vi "TurnApprox.vi"(10 "Angle":dbl, 11 "RobotDriveDevRef":T1={"DevStatus"={"status"=FALSE, "code"=0, "source"=""}, "Motors[]"=[], "Square Inputs"=FALSE, "Max Output"=1.0}) -> (3 "RobotDriveDevRef":T1={"DevStatus"={"status"=FALSE, "code"=0, "source"=""}, "Motors[]"=[], "Square Inputs"=FALSE, "Max Output"=1.0})   [LabVIEW 2016]
uses:
  <vilib>/Rock Robotics/WPI/RobotDrive/WPI_RobotDriveDevRef.ctl
  <vilib>/Rock Robotics/WPI/MotorControl/WPI_MotorControlDeviceRef.ctl
  <vilib>/Rock Robotics/WPI/MotorControl/WPI_MotorControlType.ctl
  <vilib>/Rock Robotics/SystemInterfaces/DIO/FPGA_DIOPWMChannel.ctl
  <vilib>/Rock Robotics/WPI/PWM/WPI_PWMDeadband.ctl
  Robot Global Data.vi
  <vilib>/Rock Robotics/WPI/RobotDrive/WPI_RobotDriveArcadeDrive_Standard(NoSaturation).vi
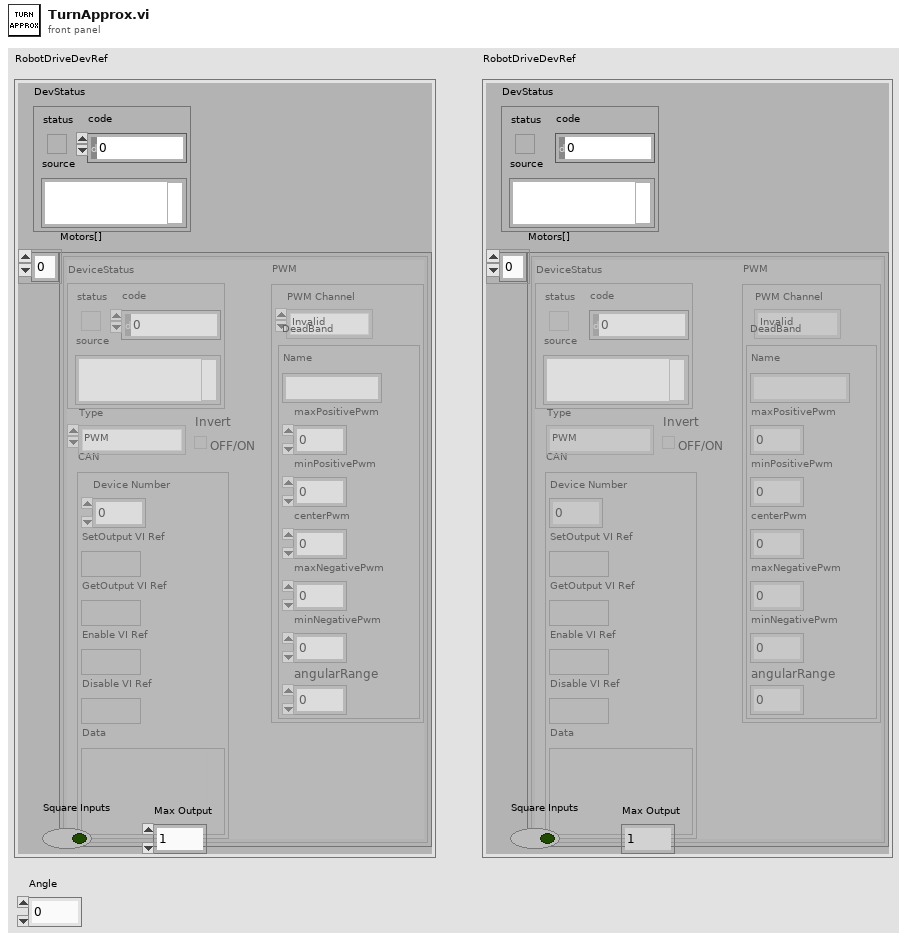
[diagram p1: front panel]
types:
  T1 = typedef "WPI_RobotDriveDevRef.ctl" = cluster{"DevStatus":errorcluster, "Motors[]":T2[], "Square Inputs":bool, "Max Output":dbl}
  T2 = typedef "WPI_MotorControlDeviceRef.ctl" = cluster{"DeviceStatus":errorcluster, "Type":T3, "PWM":cluster{"PWM Channel":T4, "DeadBand":T5}, "CAN":cluster{"Device Number":u8, "SetOutput VI Ref":variant, "GetOutput VI Ref":variant, "Enable VI Ref":variant, "Disable VI Ref":variant, "Data":variant}, "Invert":bool}
  T3 = typedef "WPI_MotorControlType.ctl" = enum16{"PWM", "CAN"}
  T4 = typedef "FPGA_DIOPWMChannel.ctl" = enum8{"PWM 0", "PWM 1", "PWM 2", "PWM 3", "PWM 4", "PWM 5", "PWM 6", "PWM 7", "PWM 8", "PWM 9", "PWM MXP 0", "PWM MXP 1", "PWM MXP 2", "PWM MXP 3", "PWM MXP 4", "PWM MXP 5", "PWM MXP 6", "PWM MXP 7", "PWM MXP 8", "PWM MXP 9", "Invalid"}
  T5 = typedef "WPI_PWMDeadband.ctl" = cluster{"Name":string, "maxPositivePwm":i32, "minPositivePwm":i32, "centerPwm":i32, "maxNegativePwm":i32, "minNegativePwm":i32, "angularRange":u16}
  T6 = cluster{"Lower X":dbl, "Lower Y":dbl, "Upper X":dbl, "Upper Y":dbl, "Lower Limit":dbl, "Upper Limit":dbl}
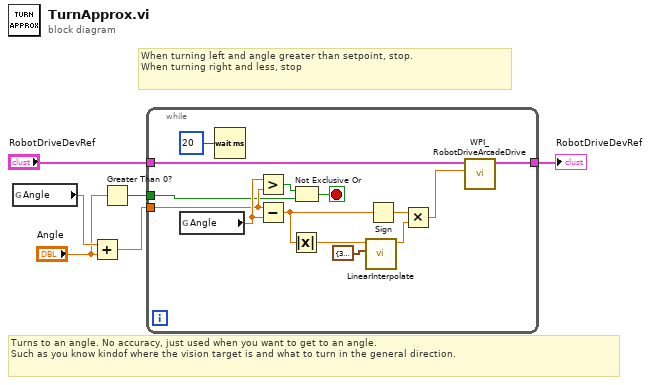
[diagram p0: block diagram]
diagram:
  # "When turning left and angle greater than setpoint, stop.\nWhen turning right and less, stop"
  # "Turns to an angle. No accuracy, just used when you want to get to an angle.\nSuch as you know kindof where the vision target is and what to turn in the general direction."
  n1 = global read "Robot Global Data.vi" "Angle"() -> (w3:dbl)
  n2 = Add(x=w3, y="Angle") -> (x+y=w4:dbl)
  n3 = Greater Than 0?(x="Angle") -> (x > 0?=w1:bool)
  n4 = while {
    tunnel: "RobotDriveDevRef" -> [w20]
    tunnel: [w19] -> w5
    tunnel: w4 -> [w10]
    tunnel: w1 -> [w8]
    stop <- w7 stop-if-true
    n5 = global read "Robot Global Data.vi" "Angle"() -> (w11:dbl)
    n6 = Wait (ms)(milliseconds to wait=u32 20) -> ()  [unwired: 1 out]
    n7 = Greater?(x=w11, y=w10) -> (0:w9:bool)
    n8 = Subtract(x=w10, y=w11) -> (x-y=w15:dbl)
    n9 = Absolute Value(x=w15) -> (abs(x)=w16:dbl)
    n10 = Not Exclusive Or(1:w8, 2:w9) -> (0:w7:bool)
    n11 = call "LinearInterpolate.vi"("Config"=T6 {"Lower X"=30.0, "Lower Y"=0.55, "Upper X"=100.0, "Upper Y"=0.9, "Lower Limit"=0.6, "Upper Limit"=0.9}, "Value"=w16) -> ("Ouput"=w12:dbl)  [unwired: 9 in]
    n12 = Sign(1:w15) -> (0:w14:dbl)
    n13 = Multiply(x=w14, y=w12) -> (x*y=w13:dbl)
    n14 = call-poly <vilib>:"WPI_RobotDriveArcadeDrive.vi"("X axis value"=w13, "RobotDriveDevRef"=w20) -> ("RobotDriveDevRef"=w19:T1)  [unwired: 7 in, 2 out]
  }
  "RobotDriveDevRef" <- w5
